vi "Read Start.vi"(8 "error in (no error)":errorcluster, 9 "timeout (0)":i32, 11 "MB_TCP in":refnum<class "MB_TCP.lvclass">) -> (0 "error out":errorcluster, 1 "Stop":bool, 2 "Start":bool, 3 "MB_TCP out":refnum<class "MB_TCP.lvclass">, 4 "timed out?":bool)   [LabVIEW 2021, in "MB_TCP.lvclass"]
uses:
  MB_TCP.lvclass
  MB_TCP.lvclass/MB_TCP.ctl
  Eth Status/Eth Status.lvlib
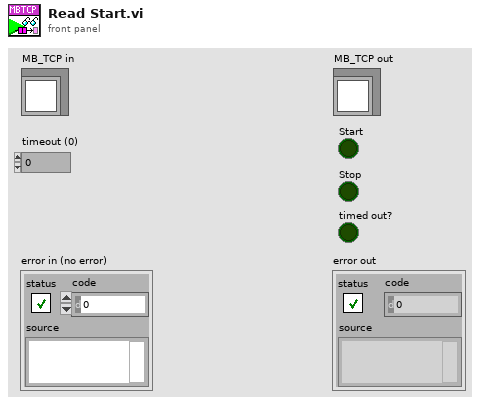
[diagram p1: front panel]
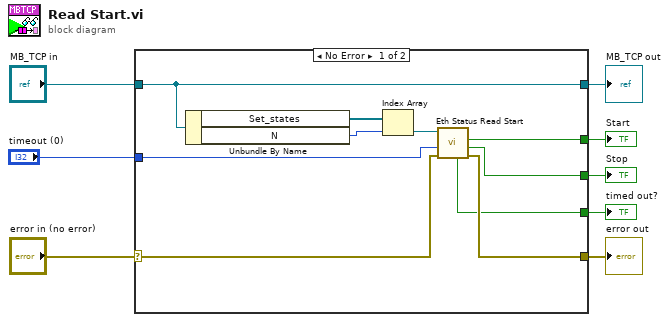
[diagram p0: block diagram]
diagram:
  n1 = case shown="No Error" "error in (no error)" {
    selector: "error in (no error)" -> [w17 w19]
    tunnel: [w16 w19] -> w7
    tunnel: [w18 w20] -> w5
    tunnel: "MB_TCP in" -> [w18 w20]
    tunnel: [w11 _] -> w4
    tunnel: "timeout (0)" -> [w12 _]
    tunnel: [w10 _] -> w2
    tunnel: [w9 _] -> w1
    frame No Error {
      n2 = Unbundle By Name(w18) -> ("Set_states"=w15:refnum<queue>[], "N"=w14:i32)
      n3 = Index Array(array=w15, index=w14) -> (element=w13:refnum<queue>)
      n4 = call "Eth Status Read Start.vi"("error in (no error)"=w17, "timeout (0)"=w12, "Set_state"=w13) -> ("error out"=w16:errorcluster, "Stop"=w10:bool, "Start"=w11:bool, "timed out?"=w9:bool)  [unwired: 4 in, 1 out]
    }
    frame Error {
    }
  }
  "error out" <- w7
  "MB_TCP out" <- w5
  "Start" <- w4
  "Stop" <- w2
  "timed out?" <- w1
